vi "Create UI Display.vi"(8 "error in (no error)":errorcluster, 10 "UI Display":refnum<vi>, 11 "References in":T1) -> (0 "error out":errorcluster, 3 "References out":T1)   [LabVIEW 2021, in "Build Script Common.lvlib"]
uses:
  Typedef/References.ctl
  Build Script Common.lvlib
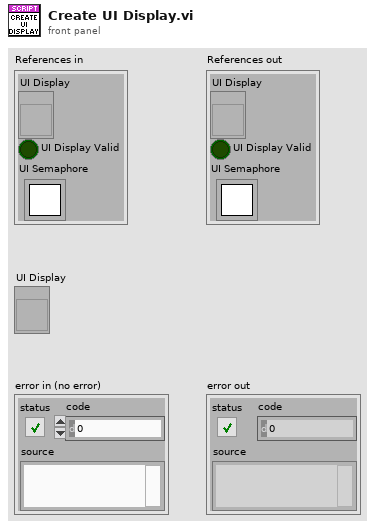
[diagram p1: front panel]
types:
  T1 = typedef "Build Script Common.lvlib/References.ctl" = cluster{"UI Display":refnum<vi>, "UI Display Valid":bool, "UI Semaphore":T2}
  T2 = typedef "Semaphore RefNum" = refnum<k1>
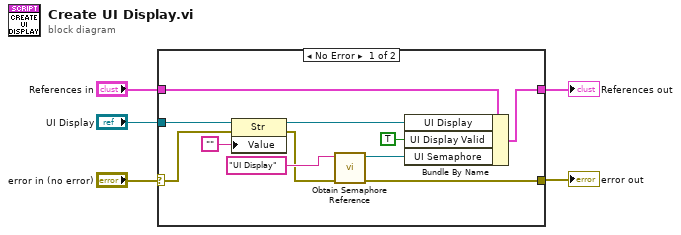
[diagram p0: block diagram]
diagram:
  n1 = case shown="No Error" "error in (no error)" {
    selector: "error in (no error)" -> [w8 w18]
    tunnel: "References in" -> [w16 w17]
    tunnel: "UI Display" -> [w10 _]
    tunnel: [w15 w17] -> w3
    tunnel: [w11 w18] -> w1
    frame No Error {
      n2 = property class="Str"(reference=w10, error in=w8, "Value"="") -> (reference out=w9:refnum<vi>, error out=w7:errorcluster)
      n3 = call <vilib>:"Obtain Semaphore Reference.vi"("error in (no error)"=w7, "name (unnamed)"="UI Display") -> ("error out"=w11:errorcluster, "semaphore"=w13:T2)  [unwired: 3 in, 1 out]
      n4 = Bundle By Name(cluster=w16, "UI Display"=w9, "UI Display Valid"=TRUE, "UI Semaphore"=w13) -> (w15:T1)
    }
    frame Error {
    }
  }
  "References out" <- w3
  "error out" <- w1
